vi "数据查询_校准记录.vi"() -> ()   [LabVIEW 2016]
uses:
  <vilib>/Utility/miscctls.llb/LVPointTypeDef.ctl
  <vilib>/Utility/miscctls.llb/LVRowAndColumnUnsignedTypeDef.ctl
  <userlib>/_OpenG.lib/array/array.llb/Remove Duplicates from 1D Array (String)__ogtk.vi
  <userlib>/_OpenG.lib/array/array.llb/Sort 2D Array (String)__ogtk.vi
  <vilib>/addons/database/_DB Variant To Data/Database Variant To Data.xnode
panel:
  in  "页":i32 format="第%.0f页"
  in  "每页条数":i32=1000
  in  "向后按钮":bool
  in  "向前按钮":bool
  in  "下拉列表":string(xcontrol)
  in  "导出":bool
  in  "查询":bool
  in  "结束日期":string="2050/01/01"
  in  "起始日期":string="2010/01/01"
  out "数据表":string[][](table)
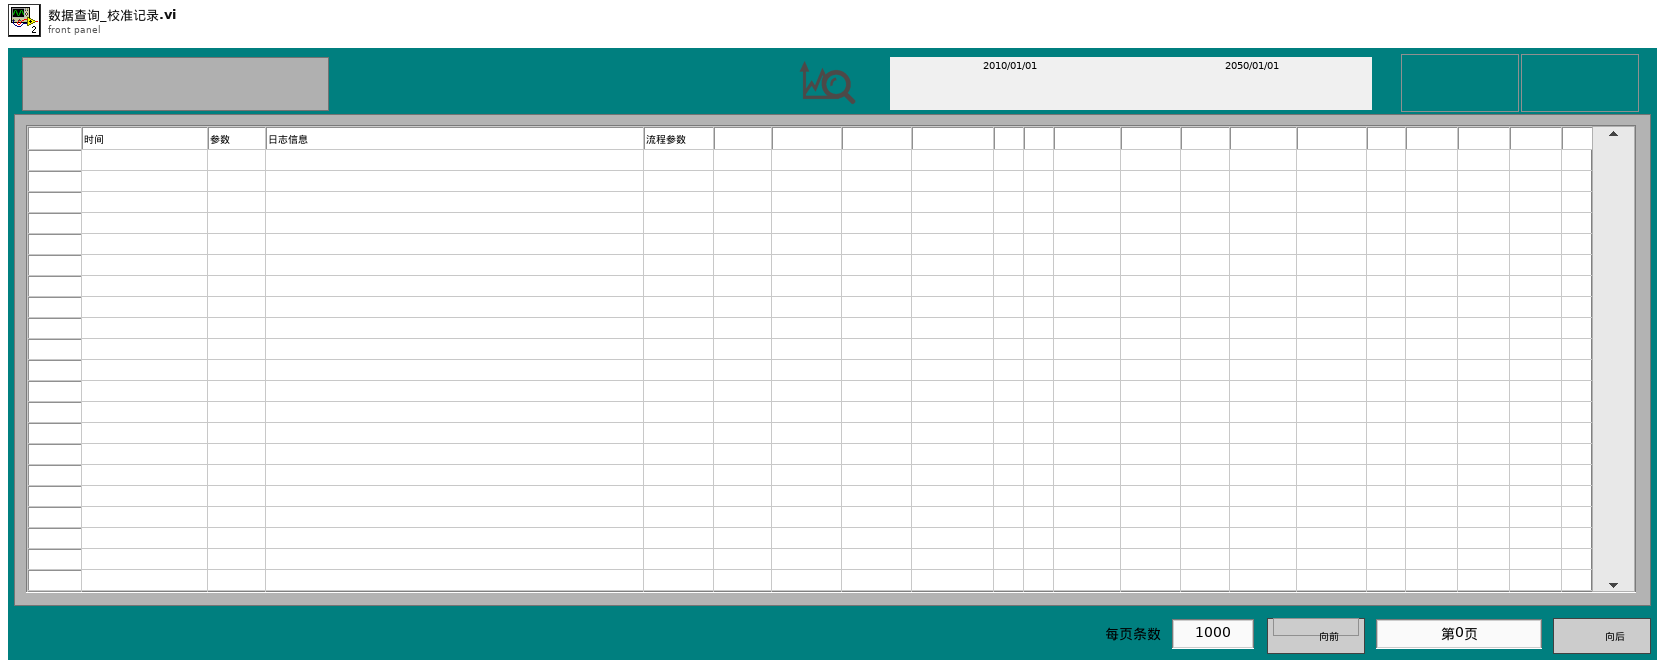
[diagram p1: front panel]
types:
  T1 = typedef "LVPointTypeDef.ctl" = cluster{"Horizontal":i16, "Vertical":i16}
  T2 = typedef "LVDateTimeRec.ctl" = cluster{"秒数的小数部分":dbl, "秒":i32, "分":i32, "时":i32, "日":i32, "月":i32, "年":i32, "天数（周）":i32, "天数（年）":i32, "DST":i32}
  T3 = enum8{"Enabled", "Disabled", "Disabled and Grayed Out"}
  T4 = typedef "LVRowAndColumnUnsignedTypeDef.ctl" = cluster{"Row":u32, "Column":u32}
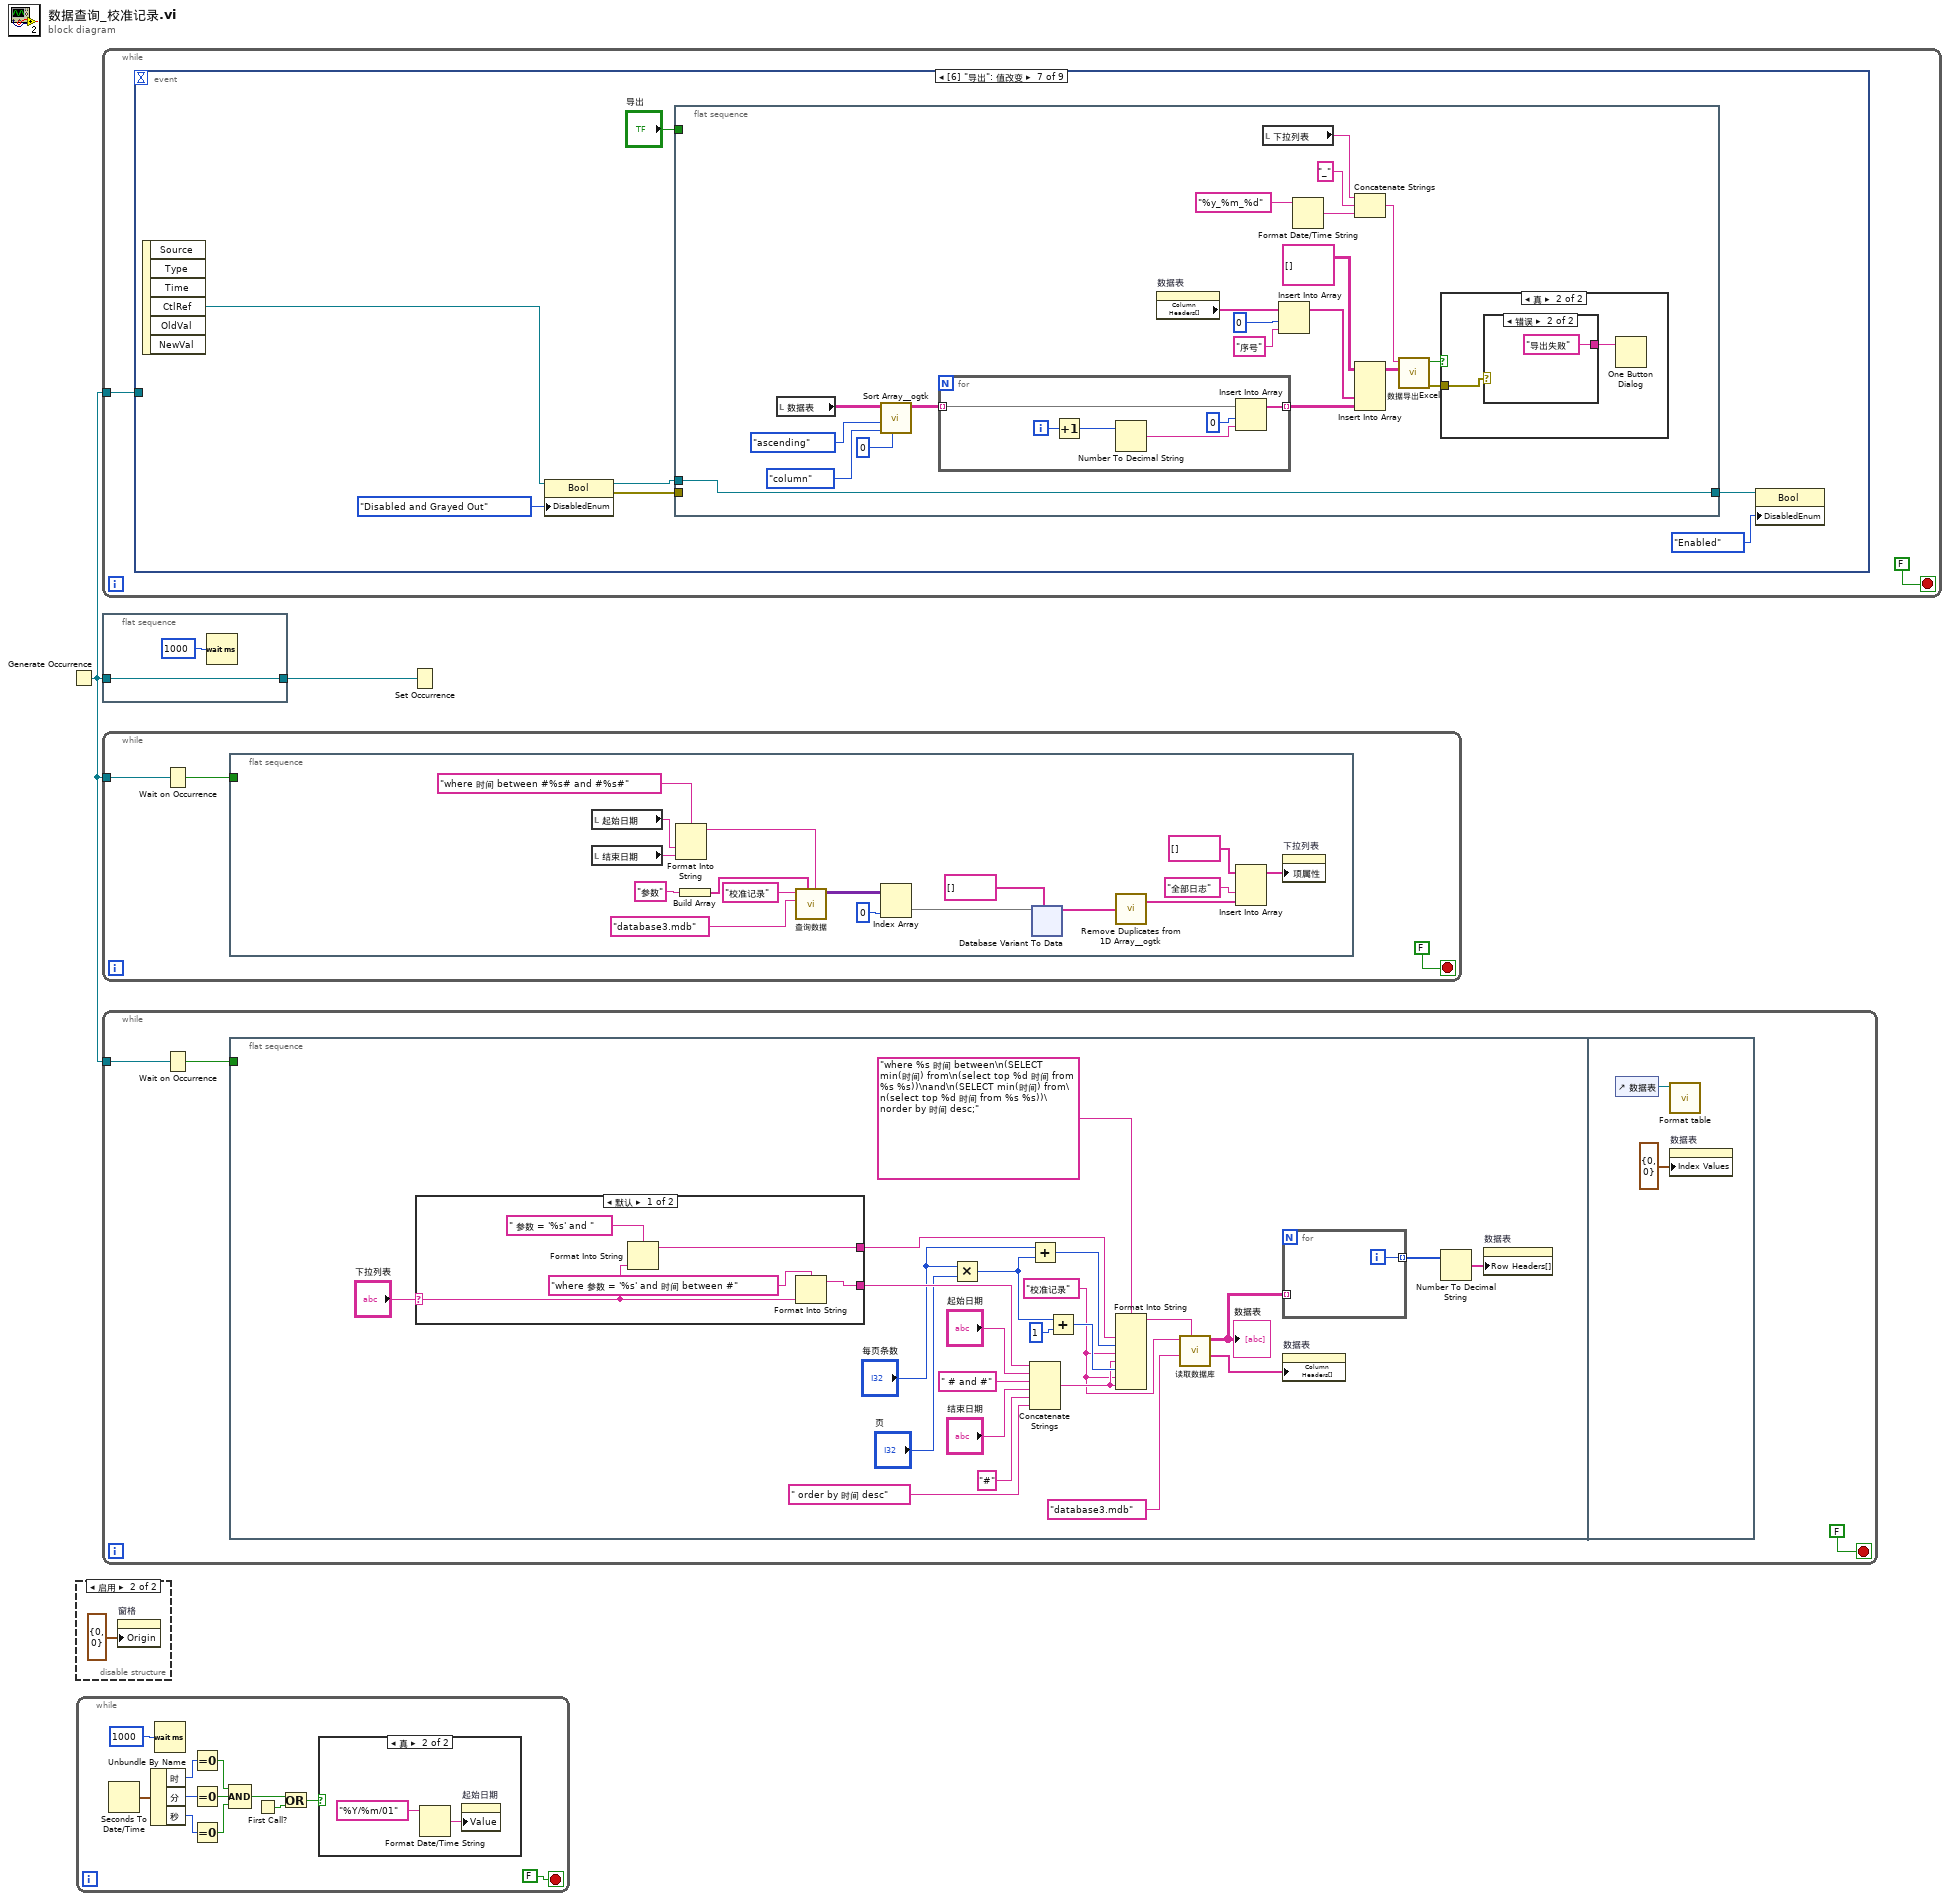
[diagram p0: block diagram]
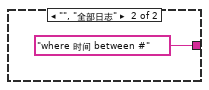
[diagram p2: hidden frame]
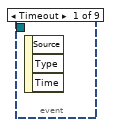
[diagram p4: hidden frame]
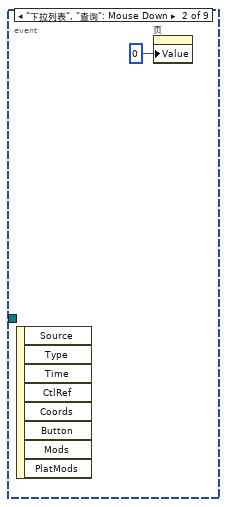
[diagram p5: hidden frame]
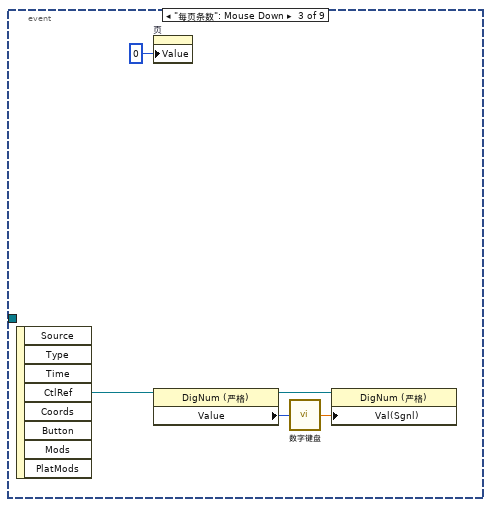
[diagram p6: hidden frame]
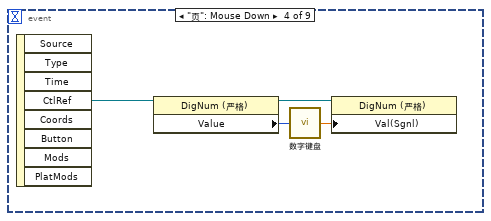
[diagram p7: hidden frame]
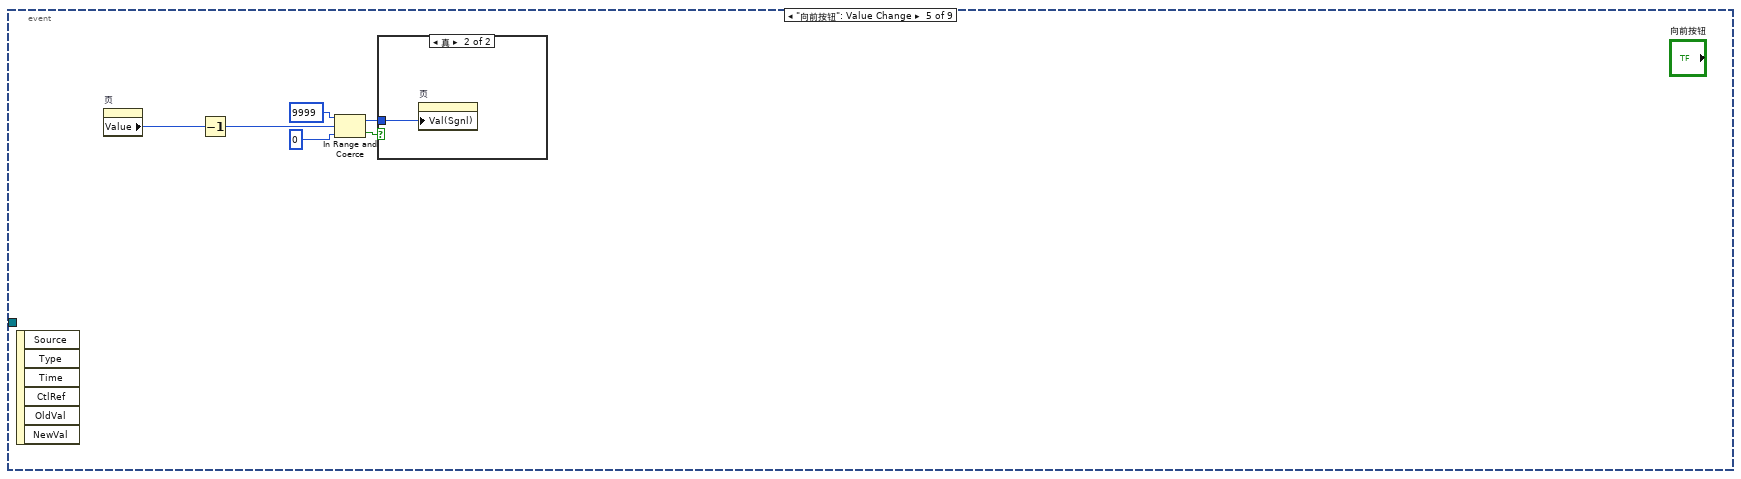
[diagram p8: hidden frame]
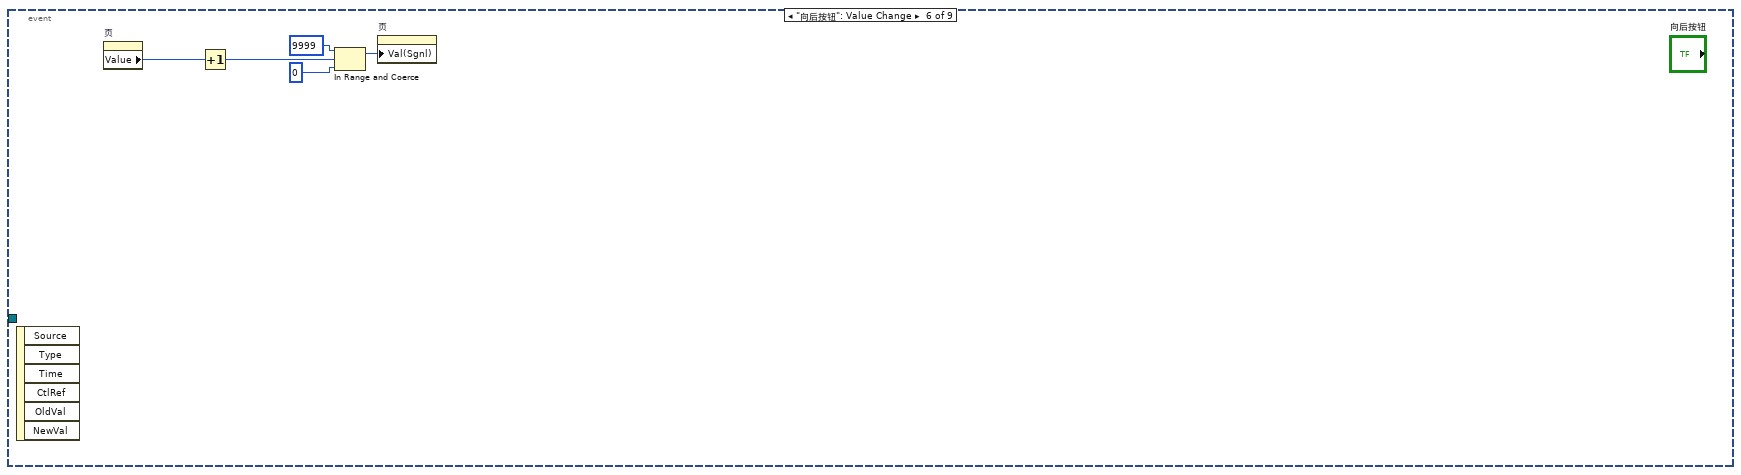
[diagram p10: hidden frame]
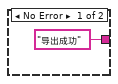
[diagram p12: hidden frame]
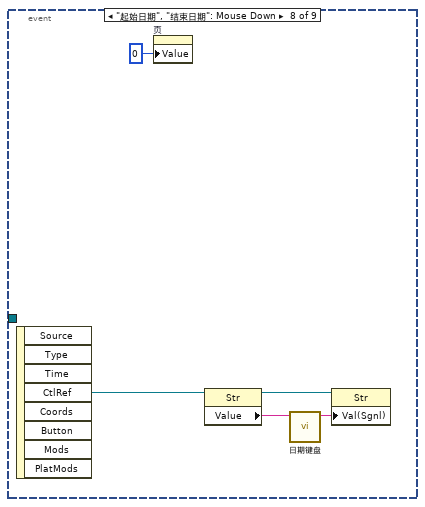
[diagram p13: hidden frame]
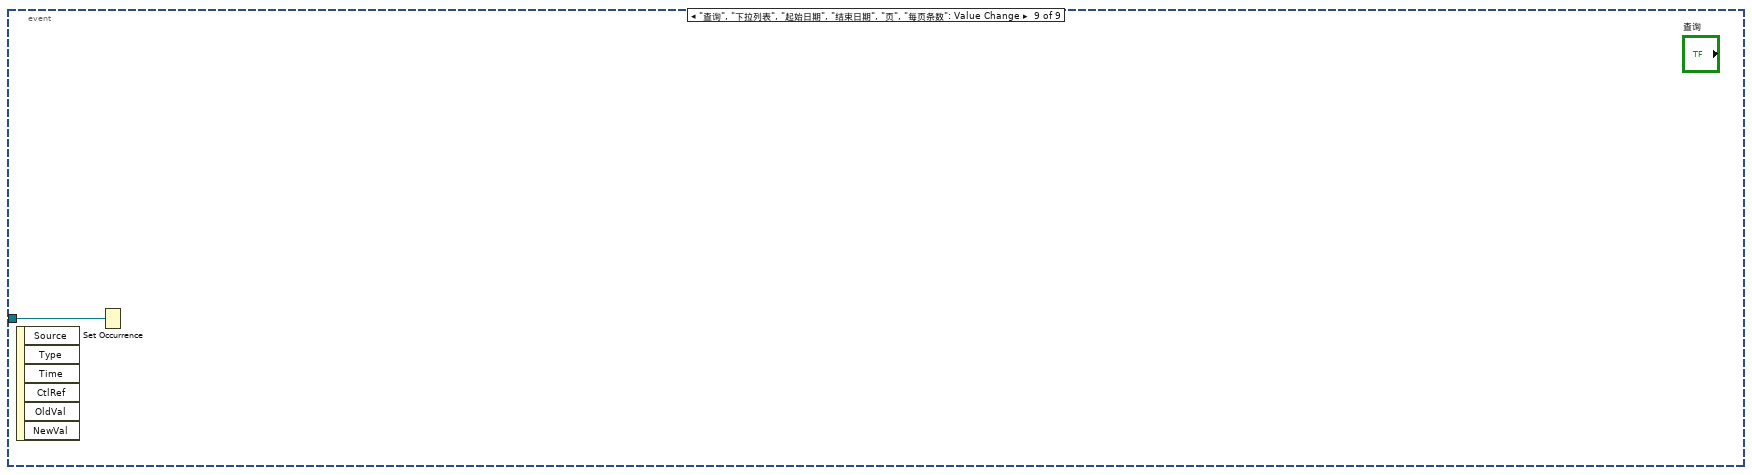
[diagram p14: hidden frame]
diagram:
  n1 = Generate Occurrence() -> (w2:refnum<k4>)
  n2 = disable-structure shown="启用" {
    frame Disabled {
    }
    frame Enabled {
      n3 = property on="窗格" class="Pane"("Origin"=T1 {"Horizontal"=0, "Vertical"=0} ("原点")) -> ()  [unwired: 2 in, 2 out]
    }
  }
  n4 = while {
    stop <- FALSE stop-if-true
    n5 = Seconds To Date/Time() -> (date time rec=w15:T2)  [unwired: 2 in]
    n6 = Unbundle By Name(w15) -> ("时"=w14:i32, "分"=w13:i32, "秒"=w12:i32)
    n7 = Wait (ms)(milliseconds to wait=u32 1000 ("等待时间（毫秒）")) -> ()  [unwired: 1 out]
    n8 = Equal To 0?(x=w14) -> (x = 0?=w11:bool)
    n9 = Equal To 0?(x=w13) -> (x = 0?=w10:bool)
    n10 = Equal To 0?(x=w12) -> (x = 0?=w9:bool)
    n11 = Compound Arithmetic op=AND ("复合运算")(w11, w10, w9) -> (w6:bool)
    n12 = First Call?() -> (First Call?: T/F=w4:bool)
    n13 = Or(x=w6, y=w4) -> (x .or. y?=w5:bool)
    n14 = case shown="真" w5 {
      frame False {
      }
      frame True {
        n15 = Format Date/Time String(time format string (%c)="%Y/%m/01" ("时间格式字符串(%c)")) -> (date/time string=w16:string)  [unwired: 2 in]
        n16 = property on="起始日期" class="Str"("Value"=w16) -> ()  [unwired: 2 in, 2 out]
      }
    }
  }
  n17 = while {
    tunnel: w2 -> [w18]
    stop <- FALSE stop-if-true
    n18 = event shown="[6] \"导出\": 值改变" {
      selector: _ -> [_ _ _ _ _ _ _ _ _]
      dyn-events: _ -> [_ _ _ _ _ _ _ _ _]
      timeout: _ -> [_ _ _ _ _ _ _ _ _]
      tunnel: w18 -> [_ _ _ _ _ _ _ _ w84]
      event Timeout {
        n19 = event-data() -> ()  [unwired: 1 in, 3 out]
      }
      event "下拉列表", "查询": Mouse Down {
        n20 = event-data() -> ()  [unwired: 1 in, 8 out]
        n21 = property on="页" class="DigNum (严格)"("Value"=0 ("页")) -> ()  [unwired: 2 in, 2 out]
      }
      event "每页条数": Mouse Down {
        n22 = event-data() -> ("CtlRef"=w22:refnum<vi>)  [unwired: 1 in, 7 out]
        n23 = property on="页" class="DigNum (严格)"("Value"=0 ("页")) -> ()  [unwired: 2 in, 2 out]
        n24 = property class="DigNum (严格)"(reference=w22) -> (reference out=w23:refnum<vi>, "Value"=w25:i32)  [unwired: 1 in, 1 out]
        n25 = call "数字键盘.vi"("OldNumber"=w25) -> ("NewNumber"=w24:sgl)
        n26 = property class="DigNum (严格)"(reference=w23, "Val(Sgnl)"=w24) -> ()  [unwired: 1 in, 2 out]
      }
      event "页": Mouse Down {
        n27 = event-data() -> ("CtlRef"=w26:refnum<vi>)  [unwired: 1 in, 7 out]
        n28 = property class="DigNum (严格)"(reference=w26) -> (reference out=w27:refnum<vi>, "Value"=w29:i32)  [unwired: 1 in, 1 out]
        n29 = call "数字键盘.vi"("OldNumber"=w29) -> ("NewNumber"=w28:sgl)
        n30 = property class="DigNum (严格)"(reference=w27, "Val(Sgnl)"=w28) -> ()  [unwired: 1 in, 2 out]
      }
      event "向前按钮": Value Change {
        n31 = event-data() -> ()  [unwired: 1 in, 6 out]
        n32 = property on="页" class="DigNum (严格)"() -> ("Value"=w35:i32)  [unwired: 2 in, 2 out]
        n33 = Decrement(x=w35) -> (x-1=w34:i32)
        n34 = In Range and Coerce(upper limit=9999 ("上限"), x=w34, lower limit=0 ("下限")) -> (coerced(x)=w31:i32, In Range?=w30:bool)
        n35 = case shown="真" w30 {
          tunnel: w31 -> [_ w36]
          frame False {
          }
          frame True {
            n36 = property on="页" class="DigNum (严格)"("Val(Sgnl)"=w36) -> ()  [unwired: 2 in, 2 out]
          }
        }
      }
      event "向后按钮": Value Change {
        n37 = event-data() -> ()  [unwired: 1 in, 6 out]
        n38 = property on="页" class="DigNum (严格)"() -> ("Value"=w41:i32)  [unwired: 2 in, 2 out]
        n39 = Increment(x=w41) -> (x+1=w40:i32)
        n40 = In Range and Coerce(upper limit=u32 9999 ("上限"), x=w40, lower limit=u32 0 ("下限")) -> (coerced(x)=w37:u32)  [unwired: 1 out]
        n41 = property on="页" class="DigNum (严格)"("Val(Sgnl)"=w37) -> ()  [unwired: 2 in, 2 out]
      }
      event "导出": Value Change {
        n42 = event-data() -> ("CtlRef"=w42:refnum<vi>)  [unwired: 1 in, 5 out]
        n43 = property class="Bool"(reference=w42, "DisabledEnum"=T3."Disabled and Grayed Out" ("禁用")) -> (reference out=w46:refnum<vi>, error out=w47:errorcluster)  [unwired: 1 in]
        n44 = flat-sequence {
          tunnel: w47 -> [_]
          tunnel: [w64] -> w45
          tunnel: w46 -> [w64]
          tunnel: "导出" -> [_]
          frame #0 {
            n45 = local read "数据表"() -> (w68:string[][])
            n46 = call-poly <userlib>:"Sort Array__ogtk.vi"("Column/Row to Sort By"=u32 0, "Sort By in"=enum16{"row", "column"}."column", "Order"=enum16{"ascending", "descending"}."ascending", "Array in"=w68) -> ("Sorted Array out"=w51:string[][])  [unwired: 4 in, 3 out]
            n47 = for {
              tunnel: w51 -> [w77] mode=indexing
              tunnel: [w76] -> w55 mode=indexing
              i -> [w78]
              n48 = Increment(x=w78) -> (x+1=w74:i32)
              n49 = Number To Decimal String(number=w74) -> (decimal integer string=w73:string)  [unwired: 1 in]
              n50 = Insert Into Array(array=w77, index=0 ("索引"), new element=w73) -> (w76:string[])
            }
            n51 = property on="数据表" class="Tbl (严格)"() -> ("Column Headers[]"=w58:string[])  [unwired: 2 in, 2 out]
            n52 = local read "下拉列表"() -> (w50:string)
            n53 = Insert Into Array(array=w58, index=0 ("索引"), new element="序号" ("新元素/子数组")) -> (w59:string[])
            n54 = Format Date/Time String(time format string (%c)="%y_%m_%d" ("时间格式字符串(%c)")) -> (date/time string=w61:string)  [unwired: 2 in]
            n55 = Concatenate Strings(w50, "_" ("字符串"), w61) -> (w60:string)
            n56 = Insert Into Array(array=string[][] [], new element #1=w59, new element #2=w55) -> (w54:string[][])  [unwired: 2 in]
            n57 = call "数据导出Excel.vi"("text data"=w54, "default name"=w60) -> ("error out"=w53:errorcluster, "布尔"=w52:bool)  [unwired: 8 in]
            n58 = case shown="真" w52 {
              tunnel: w53 -> [_ w70]
              frame False {
              }
              frame True {
                n59 = case shown="错误" w70 {
                  tunnel: ["导出成功" ("消息") "导出失败" ("消息")] -> w69
                  frame No Error {
                  }
                  frame Error {
                  }
                }
                n60 = One Button Dialog(message=w69) -> ()  [unwired: 1 in, 1 out]
              }
            }
          }
        }
        n61 = property class="Bool"(reference=w45, "DisabledEnum"=T3."Enabled" ("禁用")) -> ()  [unwired: 1 in, 2 out]
      }
      event "起始日期", "结束日期": Mouse Down {
        n62 = event-data() -> ("CtlRef"=w83:refnum<vi>)  [unwired: 1 in, 7 out]
        n63 = property on="页" class="DigNum (严格)"("Value"=0 ("页")) -> ()  [unwired: 2 in, 2 out]
        n64 = property class="Str"(reference=w83) -> (reference out=w81:refnum<vi>, "Value"=w82:string)  [unwired: 1 in, 1 out]
        n65 = call "日期键盘.vi"("原值"=w82) -> ("x+y"=w80:string)  [unwired: 10 in]
        n66 = property class="Str"(reference=w81, "Val(Sgnl)"=w80) -> ()  [unwired: 1 in, 2 out]
      }
      event "查询", "下拉列表", "起始日期", "结束日期", "页", "每页条数": Value Change {
        n67 = event-data() -> ()  [unwired: 1 in, 6 out]
        n68 = Set Occurrence(w84) -> ()
      }
    }
  }
  n69 = flat-sequence {
    tunnel: w2 -> [w86]
    tunnel: [w86] -> w1
    frame #0 {
      n70 = Wait (ms)(milliseconds to wait=u32 1000 ("等待时间（毫秒）")) -> ()  [unwired: 1 out]
    }
  }
  n71 = while {
    tunnel: w2 -> [w87]
    stop <- FALSE stop-if-true
    n72 = Wait on Occurrence(2:w87) -> (0:w88:bool)  [unwired: 2 in]
    n73 = flat-sequence {
      tunnel: w88 -> [_]
      frame #0 {
        n74 = local read "起始日期"() -> (w91:string)
        n75 = local read "结束日期"() -> (w90:string)
        n76 = Format Into String(format string="where 时间 between #%s# and #%s#" ("格式字符串"), w91, w90) -> (resulting string=w92:string)  [unwired: 2 in, 1 out]
        n77 = Build Array("参数") -> (w100:string[])
        n78 = call "查询数据.vi"("condition"=w92, "columns"=w100, "database"="database3.mdb", "table"="校准记录") -> ("data"=w99:variant[][])  [unwired: 6 in, 1 out]
        n79 = Index Array(array=w99, index (col)=0 ("禁用的索引 (列)")) -> (element=w98:variant[])  [unwired: 1 in]
        n80 = xnode "Database Variant To Data"("database variant"=w98, "type"=string[] []) -> ("data"=w95:string[])  [unwired: 1 in, 1 out]
        n81 = call-poly <userlib>:"Remove Duplicates from 1D Array__ogtk.vi"("Input Array"=w95) -> ("Output Array"=w94:string[])  [unwired: 1 out]
        n82 = Insert Into Array(array=string[] [], new element #1="全部日志" ("新元素/子数组"), new element #2=w94) -> (w104:string[])  [unwired: 1 in]
        n83 = property on="下拉列表" class="下拉列表 (严格)"("项属性"=w104) -> ()  [unwired: 2 in, 2 out]
      }
    }
  }
  n84 = while {
    tunnel: w2 -> [w146]
    stop <- FALSE stop-if-true
    n85 = Wait on Occurrence(2:w146) -> (0:w145:bool)  [unwired: 2 in]
    n86 = flat-sequence {
      tunnel: w145 -> [_]
      frame #0 {
        w148 = "校准记录"
        n87 = case shown="默认" "下拉列表" {
          selector: "下拉列表" -> [w172 _]
          tunnel: [w175 "where 时间 between #" ("condition")] -> w160
          tunnel: [w171 _] -> w149
          frame Default {
            n88 = Format Into String(format string=" 参数 = '%s' and " ("condition"), w172) -> (resulting string=w171:string)  [unwired: 2 in, 1 out]
            n89 = Format Into String(format string="where 参数 = '%s' and 时间 between #" ("condition"), w172) -> (resulting string=w175:string)  [unwired: 2 in, 1 out]
          }
          frame "", "全部日志" {
          }
        }
        n90 = Multiply(x="每页条数", y="页") -> (x*y=w157:i32)
        n91 = Add(x="每页条数", y=w157) -> (x+y=w155:i32)
        n92 = Concatenate Strings(w160, "起始日期", " # and #" ("condition"), "结束日期", "#" ("condition"), " order by 时间 desc" ("字符串")) -> (w151:string)
        n93 = Add(x=w157, y=u32 1) -> (x+y=w154:u32)
        n94 = Format Into String(format string="where %s 时间 between\n(SELECT min(时间) from\n(select top %d 时间 from %s %s))\nand\n(SELECT min(时间) from\n(select top %d 时间 from %s %s))\norder by 时间 desc;" ("格式字符串"), w149, w155, w148, w151, w154, w148, w151) -> (resulting string=w150:string)  [unwired: 2 in, 1 out]
        n95 = call "读取数据库.vi"("condition"=w150, "database"="database3.mdb", "组合框"=w148) -> ("columns"=w166:string[], "表格"=w164:string[][])  [unwired: 5 in, 2 out]
        "数据表" <- w164
        n96 = for {
          tunnel: w164 -> [_] mode=indexing
          tunnel: [w177] -> w163 mode=indexing
          i -> [w177]
        }
        n97 = property on="数据表" class="Tbl (严格)"("Column Headers[]"=w166) -> ()  [unwired: 2 in, 2 out]
        n98 = Number To Decimal String(number=w163) -> (decimal integer string=w162:string[])  [unwired: 1 in]
        n99 = property on="数据表" class="Tbl (严格)"("Row Headers[]"=w162) -> ()  [unwired: 2 in, 2 out]
      }
      frame #1 {
        n100 = control-ref of="数据表"() -> (w178:refnum<vi>)
        n101 = call "Format table.vi"("Table输入"=w178) -> ()  [unwired: 11 in]
        n102 = property on="数据表" class="Tbl (严格)"("Index Values"=T4 {"Row"=0, "Column"=0} ("索引值")) -> ()  [unwired: 2 in, 2 out]
      }
    }
  }
  n103 = Set Occurrence(w1) -> ()
